vi "NewPath.vi"(8 "error (in)":errorcluster, 10 "Initial String":string, 11 "Markers in":string[][](array[string])) -> (0 "error (out)":errorcluster, 1 "Waypoint Array":cluster{"Latitude":dbl, "Longitude":dbl}[](array[cluster]), 2 "Balloon":string, 3 "Markers out":string[][](array[string]))   [LabVIEW 2015]
uses:
  <vilib>/Utility/NIReport.llb/Append Text Table to Report (wrap).vi
  <vilib>/Utility/NIReport.llb/NI_report.lvclass
panel:
  in  "Character":string(combo) caption="Combo Box"
  in  "Color":string(combo) caption="Combo Box"
  in  "Size":string(combo) caption="Combo Box"
  in  "Longitude":dbl caption="Numeric"
  in  "Latitude":dbl caption="Numeric"
  in  "Add Marker":bool caption="New"
  out "Marker Log":string caption="String"
  in  "Reset":bool
  in  "Abort":bool
  in  "Save":bool
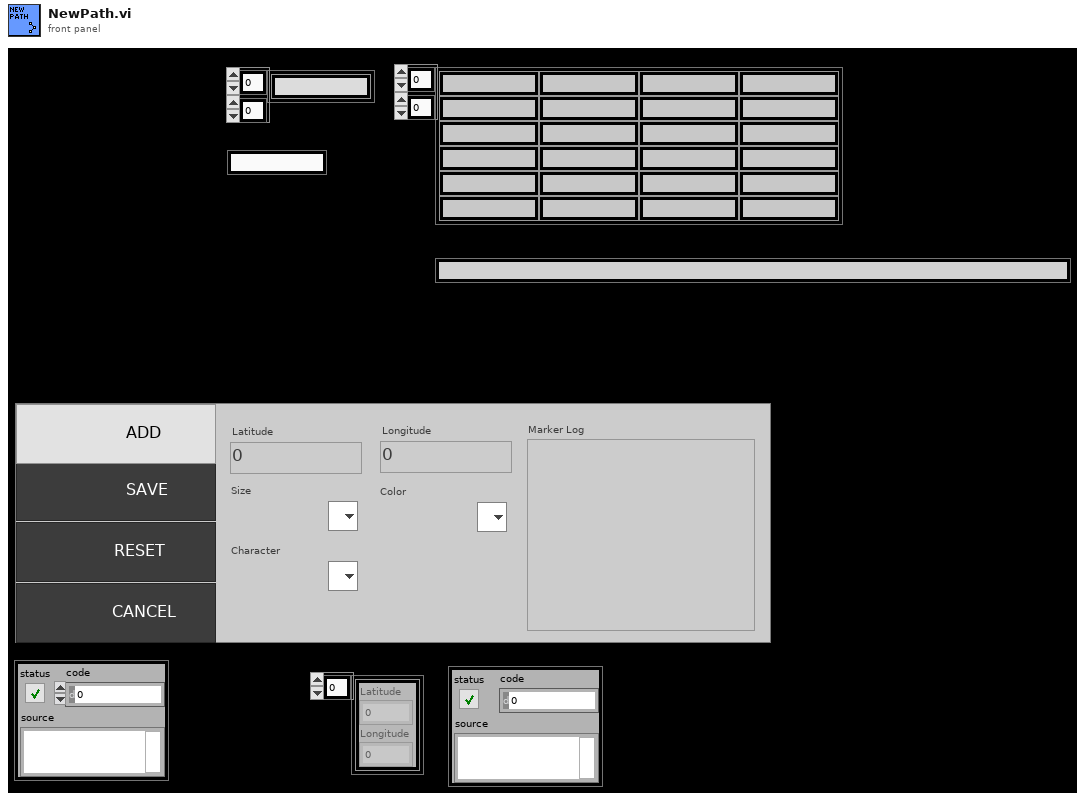
[diagram p1: front panel]
types:
  T1 = enum16{"Standard Report", "HTML", "Word", "Excel"}
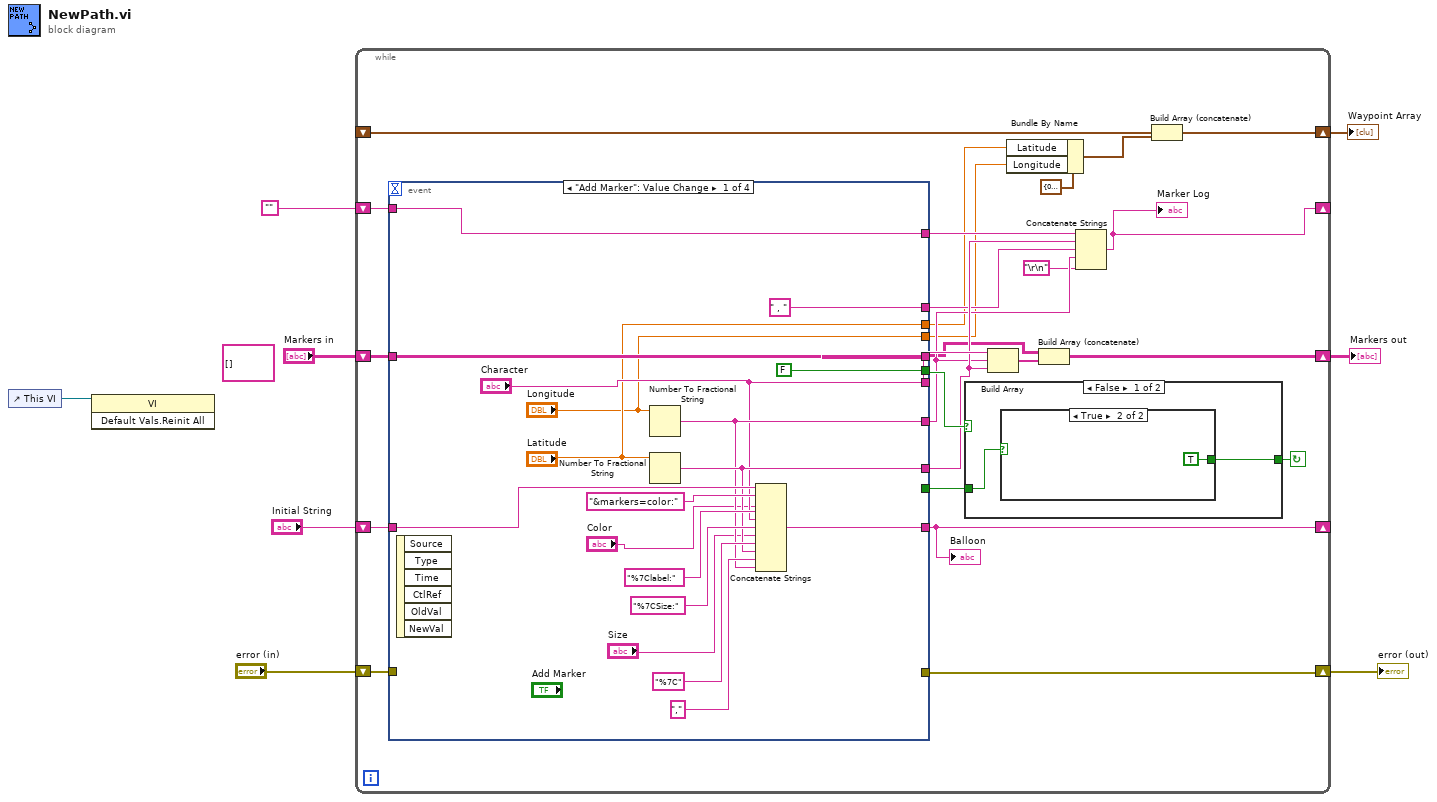
[diagram p0: block diagram]
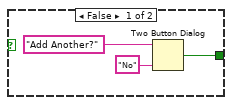
[diagram p2: hidden frame]
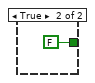
[diagram p3: hidden frame]
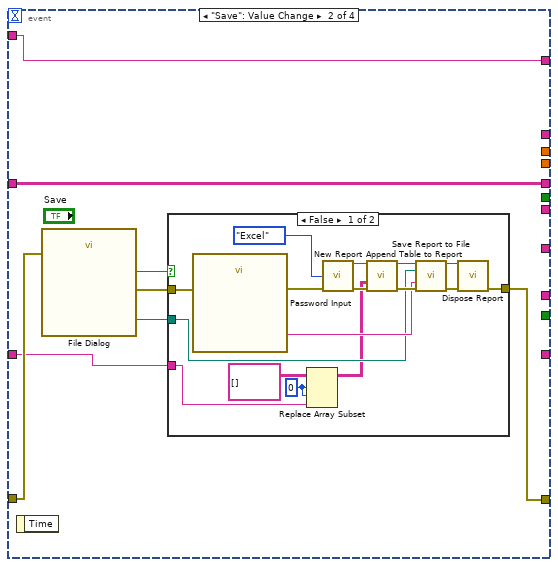
[diagram p4: hidden frame]
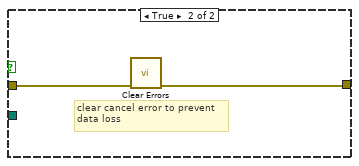
[diagram p5: hidden frame]
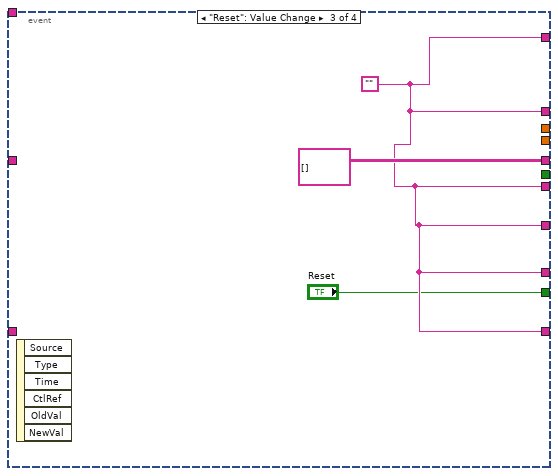
[diagram p6: hidden frame]
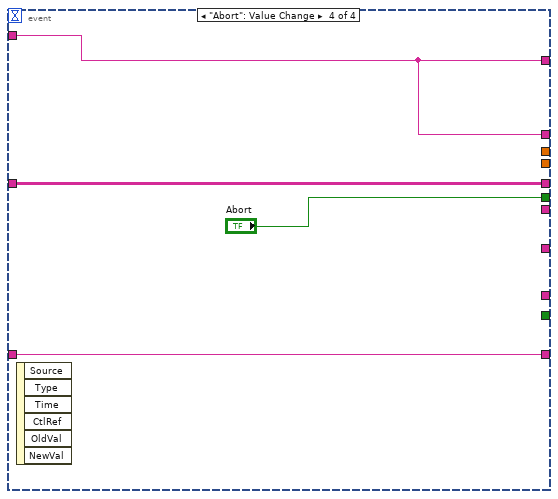
[diagram p7: hidden frame]
diagram:
  (unwired) string[][] [] ("Markers in")
  n1 = control-ref of="This VI"() -> (w4:refnum<vi>)
  n2 = invoke class="VI" method="Default Vals.Reinit All"(reference=w4) -> ()  [unwired: 2 in, 3 out]
  n3 = while {
    shift-right: [w30] -> _
    shift-left: "Initial String" -> [w33]
    shift-right: [w27] -> w7
    shift-left: "Markers in" -> [w22]
    shift-right: [w23] -> _
    shift-left: "" -> [w20]
    shift-right: [w11] -> w3
    shift-left: _ -> [w13]
    shift-right: [w9] -> w1
    shift-left: "error (in)" -> [w10]
    stop <- w32 continue-if-true
    n4 = event shown="[0] \"Add Marker\": Value Change" {
      selector: _ -> [_ _ _ _]
      dyn-events: _ -> [_ _ _ _]
      timeout: _ -> [_ _ _ _]
      tunnel: [w55 _ w86 w91] -> w30
      tunnel: w33 -> [w54 w59 _ w91]
      tunnel: [FALSE ("Cancel") _ _ "Abort"] -> w31
      tunnel: [w50 _ w86 _] -> w26
      tunnel: [w49 _ w86 _] -> w25
      tunnel: ["Character" _ w86 _] -> w29
      tunnel: w22 -> [w45 w60 _ w89]
      tunnel: [w45 w60 string[][] [] ("Markers in") w89] -> w21
      tunnel: w20 -> [w44 w61 _ w88]
      tunnel: [w44 w61 w86 w88] -> w19
      tunnel: [" , " ("string") _ w86 w88] -> w18
      tunnel: [_ _ "Reset" _] -> w17
      tunnel: ["Latitude" _ _ _] -> w16
      tunnel: ["Longitude" _ _ _] -> w15
      tunnel: w10 -> [_ w63 _ _]
      tunnel: [_ w62 _ _] -> w9
      event "Add Marker": Value Change {
        n5 = event-data() -> ()  [unwired: 1 in, 6 out]
        n6 = Number To Fractional String(number="Longitude") -> (F-format string=w49:string)  [unwired: 3 in]
        n7 = Number To Fractional String(number="Latitude") -> (F-format string=w50:string)  [unwired: 3 in]
        n8 = Concatenate Strings(w54, "&markers=color:", "Color", "%7Clabel:" ("string"), "Character", "%7CSize:" ("string"), "Size", "%7C" ("string"), w50, ",", w49) -> (w55:string)
      }
      event "Save": Value Change {
        n9 = event-data() -> ()  [unwired: 1 in, 1 out]
        n10 = call "File Dialog"("error in"=w63) -> ("selected path"=w65:path, "cancelled"=w66:bool, "error out"=w64:errorcluster)  [unwired: 11 in, 1 out]
        n11 = case shown="False" w66 {
          tunnel: w64 -> [w73 w83]
          tunnel: [w72 w84] -> w62
          tunnel: w65 -> [w71 _]
          tunnel: w59 -> [w69 _]
          frame False {
            w68 = 0 ("index (row)")
            n12 = call "Password Input"("error in (no error)"=w73) -> ("Password"=w75:string, "error out"=w74:errorcluster)  [unwired: 16 in, 1 out]
            n13 = Replace Array Subset(array=string[][] [] ("appended array"), new element=w69, index (row)=w68, index (col)=w68) -> (w67:string[][])
            n14 = call <vilib>:"New Report.vi"("report type"=T1."Excel", "error in (no error)"=w74) -> ("report out"=w82:refnum<class "NI_report.lvclass">, "error out"=w81:errorcluster)  [unwired: 12 in]
            n15 = call-poly <vilib>:"Append Table to Report.vi"("report in"=w82, "text data"=w67, "error in (no error)"=w81) -> ("report out"=w80:refnum<class "NI_report.lvclass">, "error out"=w79:errorcluster)  [unwired: 9 in, 2 out]
            n16 = call-dynamic "Save Report to File.vi"("report in"=w80, "report file path"=w71, "password (\"\")"=w75, "error in (no error)"=w79) -> ("report out"=w78:refnum<class "NI_report.lvclass">, "error out"=w77:errorcluster)  [unwired: 10 in]
            n17 = call-dynamic "Dispose Report.vi"("report in"=w78, "error in (no error)"=w77) -> ("error out"=w72:errorcluster)  [unwired: 13 in]
          }
          frame True {
            # "clear cancel error to prevent \ndata loss"
            n18 = call <vilib>:"Clear Errors.vi"("error in (no error)"=w83) -> ("error out"=w84:errorcluster)  [unwired: 5 in, 1 out]
          }
        }
      }
      event "Reset": Value Change {
        w86 = ""
        n19 = event-data() -> ()  [unwired: 1 in, 6 out]
      }
      event "Abort": Value Change {
        n20 = event-data() -> ()  [unwired: 1 in, 6 out]
      }
    }
    "Balloon" <- w30
    n21 = case shown="False" w31 {
      tunnel: [w35 FALSE ("T button?")] -> w32
      tunnel: w17 -> [w34 _]
      frame False {
        n22 = case shown="True" w34 {
          tunnel: [w38 TRUE ("T button?")] -> w35
          frame False {
            n23 = Two Button Dialog(message="Add Another?", 1:"No" ("F button name (\"Cancel\")")) -> (T button?=w38:bool)  [unwired: 1 in]
          }
          frame True {
          }
        }
      }
      frame True {
      }
    }
    n24 = Build Array(w29, w25, w26) -> (w28:string[])
    n25 = Bundle By Name(cluster=cluster{"Latitude":dbl, "Longitude":dbl} {"Latitude"=0.0, "Longitude"=0.0} ("input cluster"), "Latitude"=w16, "Longitude"=w15) -> (w12:cluster{"Latitude":dbl, "Longitude":dbl})
    n26 = Build Array (concatenate)(w21, w28) -> (w27:string[][])
    n27 = Concatenate Strings(w19, w26, w18, w25, "\r\n") -> (w23:string)
    "Marker Log" <- w23
    n28 = Build Array (concatenate)(w13, w12) -> (w11:cluster{"Latitude":dbl, "Longitude":dbl}[])
  }
  "Markers out" <- w7
  "Waypoint Array" <- w3
  "error (out)" <- w1
